vi "G1.vi"   [LabVIEW 2013]
uses:
  Global test.vi
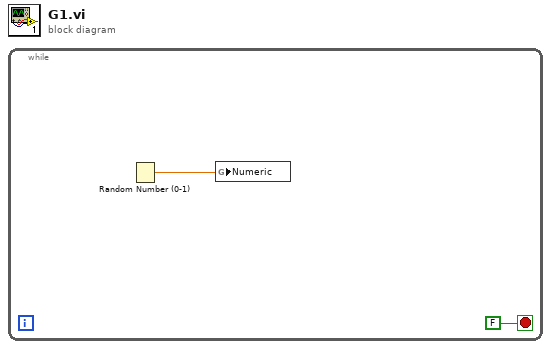
[diagram p0: block diagram]
diagram:
  n1 = while {
    stop <- FALSE stop-if-true
    n2 = Random Number (0-1)() -> (number: 0 to 1=w1:dbl)
    n3 = global write "Global test.vi" "Numeric"(w1) -> ()
  }
